vi "Return_Specific_Header.vi"(8 "error in (no error)":errorcluster, 10 "Specific Header":string, 11 "Response in":refnum<class "Response.lvclass">) -> (0 "error out":errorcluster, 2 "Value":string, 3 "Response out":refnum<class "Response.lvclass">)   [LabVIEW 2020, in "Response.lvclass"]
uses:
  Response.lvclass
  Response.lvclass/Response.ctl
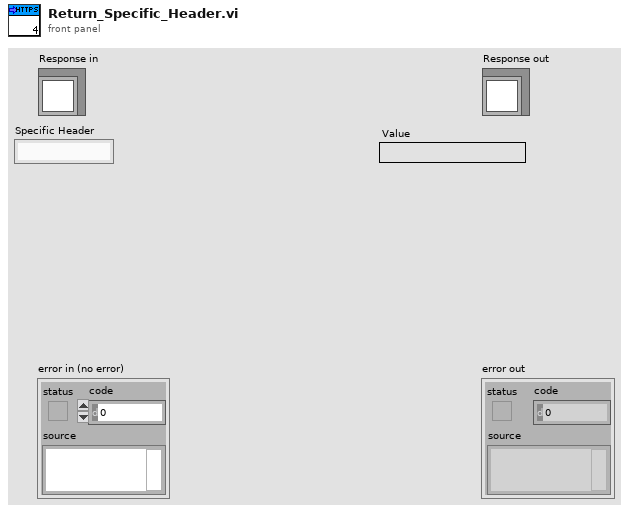
[diagram p1: front panel]
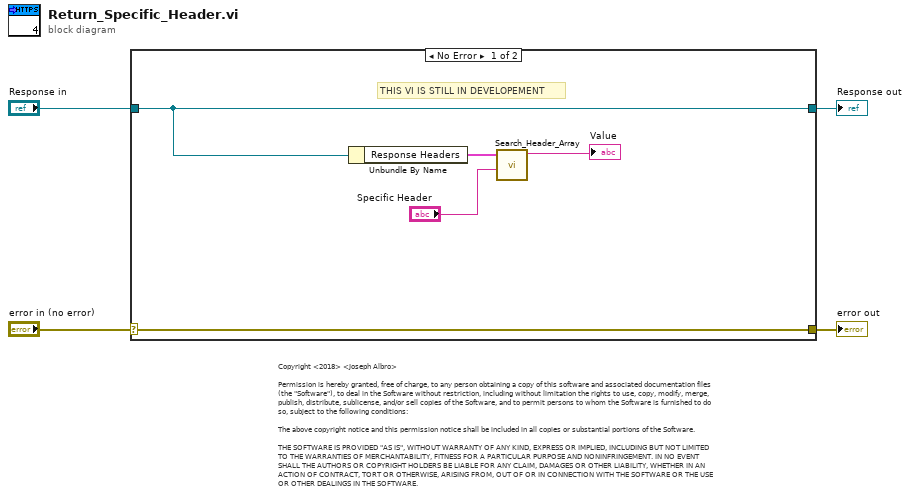
[diagram p0: block diagram]
diagram:
  # "Copyright <2018> <Joseph Albro>\n\nPermission is hereby granted, free of charge, to any person obtaining a copy of this software and associated documentation files (the \"Software\"), to deal in the Software without restriction, including without limitation the rights to use, copy, modify, merge, publish, distribute, sublicense, and/or sell copies of the Software, and to permit persons to whom the Software is furnished to do so, subject to the following conditions:\n\nThe above copyright notice and this permission notice shall be included in all copies or substantial portions of the Software.\n\nTHE SOFTWARE IS PROVIDED \"AS IS\", WITHOUT WARRANTY OF ANY KIND, EXPRESS OR IMPLIED, INCLUDING BUT NOT LIMITED TO THE WARRANTIES OF MERCHANTABILITY, FITNESS FOR A PARTICULAR PURPOSE AND NONINFRINGEMENT. IN NO EVENT SHALL THE AUTHORS OR COPYRIGHT HOLDERS BE LIABLE FOR ANY CLAIM, DAMAGES OR OTHER LIABILITY, WHETHER IN AN ACTION OF CONTRACT, TORT OR OTHERWISE, ARISING FROM, OUT OF OR IN CONNECTION WITH THE SOFTWARE OR THE USE OR OTHER DEALINGS IN THE SOFTWARE."
  n1 = case shown="No Error" "error in (no error)" {
    selector: "error in (no error)" -> [w9 w11]
    tunnel: [w9 w11] -> w3
    tunnel: [w8 w10] -> w1
    tunnel: "Response in" -> [w8 w10]
    frame No Error {
      # "THIS VI IS STILL IN DEVELOPEMENT"
      n2 = Unbundle By Name(w8) -> ("Response Headers"=w7:cluster{"Name":string, "Value":string}[])
      n3 = call "Search_Header_Array.vi"("Specific Header"="Specific Header", "Headers"=w7) -> ("Value"=→"Value":string)  [unwired: 9 in]
    }
    frame Error {
    }
  }
  "error out" <- w3
  "Response out" <- w1
